vi "Evaluation.vi"(8 "error in (no error)":errorcluster, 10 "Parents G":dbl, 11 "SudukuState in":refnum<class "SudukuState.lvclass">) -> (0 "error out":errorcluster, 1 "H":dbl, 2 "G":dbl, 3 "SudukuState out":refnum<class "SudukuState.lvclass">)   [LabVIEW 2009, in "SudukuState.lvclass"]
uses:
  SudukuState.lvclass
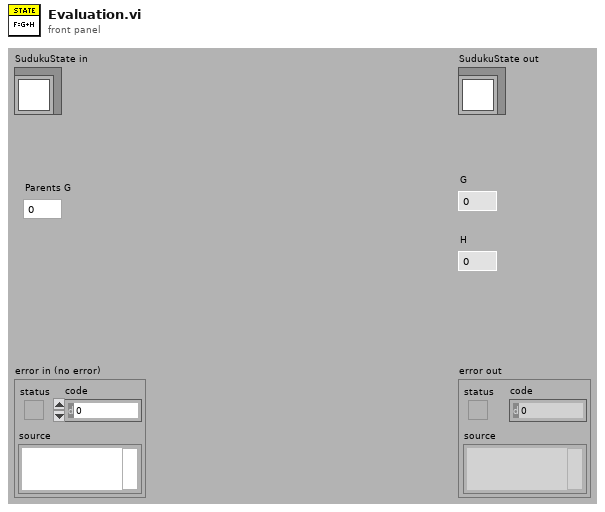
[diagram p1: front panel]
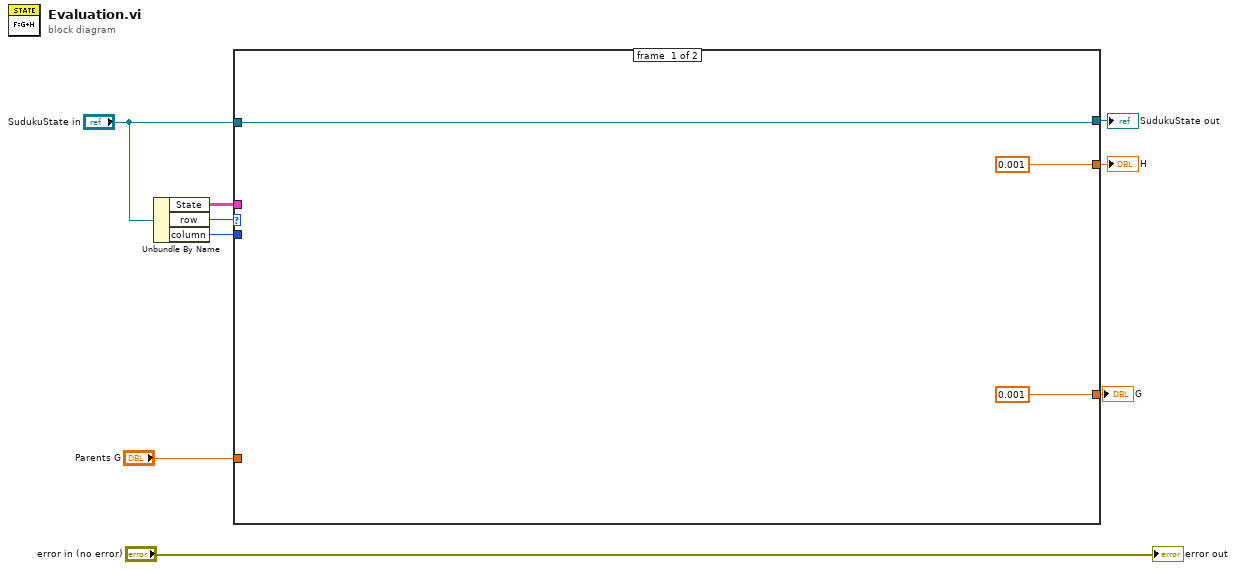
[diagram p0: block diagram]
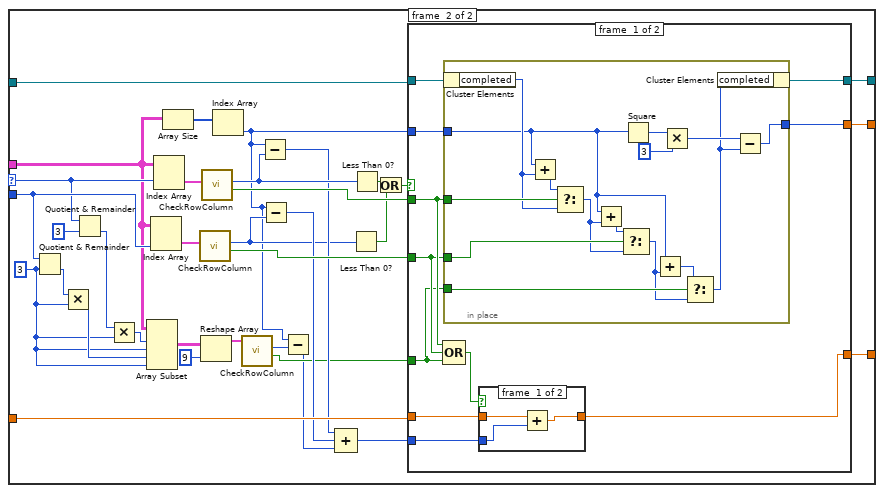
[diagram p2: hidden frame]
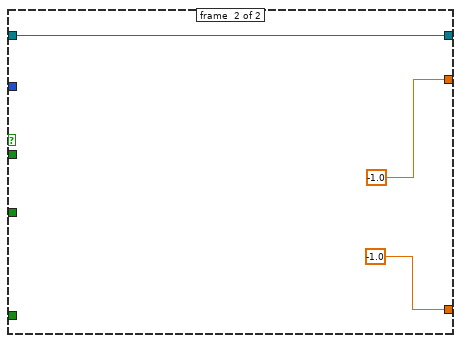
[diagram p4: hidden frame]
diagram:
  n1 = Unbundle By Name("SudukuState in") -> ("State"=w3:cluster{"Value":i32, "Options":i32[]}[][], "row"=w1:i32, "column"=w5:i32)
  n2 = case shown="Default" w1 {
    selector: w1 -> [_ w26]
    tunnel: [0.001 ("G") w45] -> w9
    tunnel: [0.001 ("G") w44] -> w8
    tunnel: "Parents G" -> [_ w42]
    tunnel: "SudukuState in" -> [w12 w41]
    tunnel: w5 -> [_ w28]
    tunnel: w3 -> [_ w25]
    tunnel: [w12 w35] -> w2
    frame #0 {
    }
    frame #1 {
      w21 = 3 ("y")
      n3 = Quotient & Remainder(x=w28, y=w21) -> (floor(x/y)=w24:i32)  [unwired: 1 out]
      n4 = Multiply(x=w24, y=w21) -> (x*y=w23:i32)
      n5 = Quotient & Remainder(x=w26, y=3) -> (floor(x/y)=w22:i32)  [unwired: 1 out]
      n6 = Multiply(x=w22, y=w21) -> (x*y=w20:i32)
      n7 = Array Subset(array=w25, index (row)=w20, length (row)=w21, index (col)=w23, length (col)=w21) -> (w19:cluster{"Value":i32, "Options":i32[]}[][])
      n8 = Index Array(array=w25, index (col)=w28) -> (element=w40:cluster{"Value":i32, "Options":i32[]}[])  [unwired: 1 in]
      n9 = Index Array(array=w25, index (row)=w26) -> (element=w46:cluster{"Value":i32, "Options":i32[]}[])  [unwired: 1 in]
      n10 = Array Size(array=w25) -> (size(s)=w36:i32[])
      n11 = call "CheckRowColumn.vi"("RowColumn"=w40) -> ("Complete"=w34:bool, "Evaluation"=w30:i32)  [unwired: 9 in]
      n12 = Reshape Array(w19, 9 ("dimension size")) -> (w17:cluster{"Value":i32, "Options":i32[]}[])
      n13 = call "CheckRowColumn.vi"("RowColumn"=w46) -> ("Complete"=w43:bool, "Evaluation"=w32:i32)  [unwired: 9 in]
      n14 = Index Array(array=w36) -> (element=w15:i32)  [unwired: 1 in]
      n15 = call "CheckRowColumn.vi"("RowColumn"=w17) -> ("Complete"=w14:bool, "Evaluation"=w16:i32)  [unwired: 9 in]
      n16 = Subtract(x=w15, y=w32) -> (x-y=w31:i32)
      n17 = Subtract(x=w15, y=w30) -> (x-y=w33:i32)
      n18 = Subtract(x=w15, y=w16) -> (x-y=w13:i32)
      n19 = Compound Arithmetic op=ADD(w31, w33, w13) -> (w29:i32)
      n20 = Less Than 0?(x=w30) -> (x < 0?=w37:bool)
      n21 = Less Than 0?(x=w32) -> (x < 0?=w39:bool)
      n22 = Or(x=w39, y=w37) -> (x .or. y?=w38:bool)
      n23 = case shown="False" w38 {
        tunnel: [w47 -1.0 ("G")] -> w45
        tunnel: [w54 -1.0 ("G")] -> w44
        tunnel: w43 -> [w53 _]
        tunnel: w42 -> [w50 _]
        tunnel: w41 -> [w57 w77]
        tunnel: [w56 w77] -> w35
        tunnel: w15 -> [w55 _]
        tunnel: w34 -> [w52 _]
        tunnel: w29 -> [w49 _]
        tunnel: w14 -> [w48 _]
        frame #0 {
          n24 = Compound Arithmetic op=OR(w53, w52, w48) -> (w51:bool)
          n25 = in-place {
            in-place-border: w53 -> [w76]
            in-place-border: w55 -> [w66]
            in-place-border: [w69] -> w54
            in-place-border: w52 -> [w68]
            in-place-border: w48 -> [w67]
            n26 = in-place-cluster #1(w57) -> ("completed"=w74:i32)
            n27 = Add(x=w66, y=w74) -> (x+y=w75:i32)
            n28 = Select(t=w75, s=w76, f=w74) -> (s? t:f=w65:i32)
            n29 = Add(x=w66, y=w65) -> (x+y=w73:i32)
            n30 = Select(t=w73, s=w68, f=w65) -> (s? t:f=w63:i32)
            n31 = Square(x=w66) -> (x^2=w72:i32)
            n32 = Add(x=w66, y=w63) -> (x+y=w64:i32)
            n33 = Multiply(x=w72, y=3) -> (x*y=w70:i32)
            n34 = Select(t=w64, s=w67, f=w63) -> (s? t:f=w62:i32)
            n35 = in-place-cluster #1("completed"=w62) -> (w56:refnum<class "SudukuState.lvclass">)
            n36 = Subtract(x=w70, y=w62) -> (x-y=w69:i32)
          }
          n37 = case shown="False" w51 {
            tunnel: [w58 w61] -> w47
            tunnel: w50 -> [w60 w61]
            tunnel: w49 -> [w59 _]
            frame #0 {
              n38 = Add(x=w60, y=w59) -> (x+y=w58:dbl)
            }
            frame #1 {
            }
          }
        }
        frame #1 {
        }
      }
    }
  }
  "SudukuState out" <- w2
  "G" <- w9
  "H" <- w8
  "error out" <- "error in (no error)"
